vi "Database.ReturnStatus.vi"(5 "repeat":bool, 7 "service":bool, 10 "Status":T1) -> (1 "skipped?":bool, 2 "Step.statusId":i32)   [LabVIEW 2016]
uses:
  Subvis/StepStatus.ctl
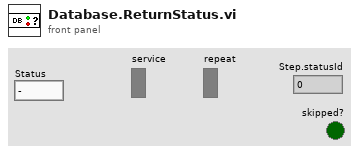
[diagram p1: front panel]
types:
  T1 = typedef "StepStatus.ctl" = enum16{"-", "Pending", "Running", "Skipped", "Passed", "Failed", "Done", "Error", "Aborted", "Stopped"}
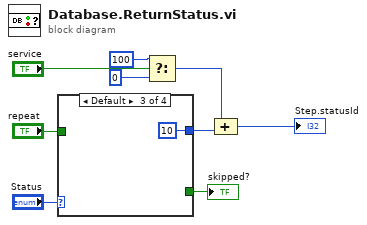
[diagram p0: block diagram]
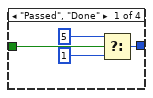
[diagram p2: hidden frame]
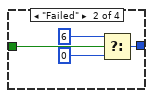
[diagram p3: hidden frame]
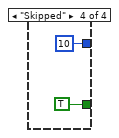
[diagram p4: hidden frame]
diagram:
  n1 = case shown="Default" "Status" {
    tunnel: "repeat" -> [w13 w17 _ _]
    tunnel: [w12 w16 10 10] -> w4
    tunnel: [_ _ _ TRUE] -> w2
    frame "Passed", "Done" {
      n2 = Select(t=5, s=w13, f=1) -> (s? t:f=w12:i32)
    }
    frame "Failed" {
      n3 = Select(t=6, s=w17, f=0) -> (s? t:f=w16:i32)
    }
    frame Default {
    }
    frame "Skipped" {
    }
  }
  "skipped?" <- w2
  n4 = Select(t=100, s="service", f=0) -> (s? t:f=w6:i32)
  n5 = Compound Arithmetic op=ADD(w6, w4) -> (→"Step.statusId":i32)
